vi "HFRR ADV v013 new software.vi"() -> ()   [LabVIEW 2025] (continued)
    n921 = Wait (ms)(milliseconds to wait=u32 20 ("millisecond timer value")) -> ()  [unwired: 1 out]
    n922 = local read "Quit"() -> (w1050:bool)
  }
  n923 = while {
    tunnel: w33 -> [_]
    tunnel: w17 -> [_]
    stop <- w1148 stop-if-true
    # "New Adv Logics"
    n924 = local read "Main Tab"() -> (w1128:T2)
    n925 = local read "Main Tab"() -> (w1146:T2)
    n926 = local read "Sign In"() -> (w1145:bool)
    n927 = case shown="\"Adv Scar\"" w1128 {
      frame "HOME", Default {
        n928 = local read "LIVE FEED MIN TEMP"() -> (w1281:bool)
        n929 = local write "LIVE FEED MAX TEMP"(TRUE ("LIVE FEED MAX TEMP")) -> ()
        n930 = local read "CAMERA ROI MIN TEMP"() -> (w1279:bool)
        n931 = case shown="True" w1281 {
          selector: w1281 -> [_ w1288]
          frame False {
          }
          frame True {
            n932 = Not(x=w1288) -> (.not. x?=w1287:bool)
            n933 = local write "LIVE FEED MIN TEMP"(w1287) -> ()
            n934 = call "CAMERA LIVE FEED FGV.vi"("Enum - Menu"=CAMERA_LIVE_FEED_ENUM."CAMERA MINIMIZE") -> ()  [unwired: 9 in, 2 out]
          }
        }
        n935 = case shown="True" w1279 {
          selector: w1279 -> [_ w1285]
          frame False {
          }
          frame True {
            n936 = Not(x=w1285) -> (.not. x?=w1284:bool)
            n937 = local write "CAMERA ROI MIN TEMP"(w1284) -> ()
            n938 = call "IMAGE ANALYSIS.vi"("Enum"=POST_ANALYSIS_ENUM."MINIMIZE UI") -> ()  [unwired: 9 in, 2 out]
          }
        }
        n939 = local write "CAMERA ROI MAX TEMP"(TRUE ("CAMERA ROI MAX TEMP")) -> ()
      }
      frame "Test Setup" {
        n940 = local read "LIVE FEED MIN TEMP"() -> (w1291:bool)
        n941 = local read "CAMERA ROI MIN TEMP"() -> (w1289:bool)
        n942 = local write "LIVE FEED MAX TEMP"(TRUE ("LIVE FEED MAX TEMP")) -> ()
        n943 = case shown="True" w1291 {
          selector: w1291 -> [_ w1298]
          frame False {
          }
          frame True {
            n944 = Not(x=w1298) -> (.not. x?=w1297:bool)
            n945 = local write "LIVE FEED MIN TEMP"(w1297) -> ()
            n946 = call "CAMERA LIVE FEED FGV.vi"("Enum - Menu"=CAMERA_LIVE_FEED_ENUM."CAMERA MINIMIZE") -> ()  [unwired: 9 in, 2 out]
          }
        }
        n947 = case shown="True" w1289 {
          selector: w1289 -> [_ w1295]
          frame False {
          }
          frame True {
            n948 = Not(x=w1295) -> (.not. x?=w1294:bool)
            n949 = local write "CAMERA ROI MIN TEMP"(w1294) -> ()
            n950 = call "IMAGE ANALYSIS.vi"("Enum"=POST_ANALYSIS_ENUM."MINIMIZE UI") -> ()  [unwired: 9 in, 2 out]
          }
        }
        n951 = local write "CAMERA ROI MAX TEMP"(TRUE ("CAMERA ROI MAX TEMP")) -> ()
      }
      frame "Acquire" {
        n952 = local read "LIVE FEED MIN TEMP"() -> (w1301:bool)
        n953 = local write "LIVE FEED MAX TEMP"(TRUE ("LIVE FEED MAX TEMP")) -> ()
        n954 = local read "CAMERA ROI MIN TEMP"() -> (w1299:bool)
        n955 = case shown="True" w1301 {
          selector: w1301 -> [_ w1308]
          frame False {
          }
          frame True {
            n956 = Not(x=w1308) -> (.not. x?=w1307:bool)
            n957 = local write "LIVE FEED MIN TEMP"(w1307) -> ()
            n958 = call "CAMERA LIVE FEED FGV.vi"("Enum - Menu"=CAMERA_LIVE_FEED_ENUM."CAMERA MINIMIZE") -> ()  [unwired: 9 in, 2 out]
          }
        }
        n959 = case shown="True" w1299 {
          selector: w1299 -> [_ w1305]
          frame False {
          }
          frame True {
            n960 = Not(x=w1305) -> (.not. x?=w1304:bool)
            n961 = local write "CAMERA ROI MIN TEMP"(w1304) -> ()
            n962 = call "IMAGE ANALYSIS.vi"("Enum"=POST_ANALYSIS_ENUM."MINIMIZE UI") -> ()  [unwired: 9 in, 2 out]
          }
        }
        n963 = local write "CAMERA ROI MAX TEMP"(TRUE ("CAMERA ROI MAX TEMP")) -> ()
      }
      frame "Adv Scar" {
        n964 = local read "CAMERA ROI MIN TEMP"() -> (w1309:bool)
        n965 = case shown="True" "LIVE FEED MAX TEMP" {
          selector: "LIVE FEED MAX TEMP" -> [_ w1330]
          frame False {
          }
          frame True {
            n966 = Not(x=w1330) -> (.not. x?=w1329:bool)
            n967 = local write "LIVE FEED MAX TEMP"(w1329) -> ()
            n968 = call "CAMERA LIVE FEED FGV.vi"("Enum - Menu"=CAMERA_LIVE_FEED_ENUM."CAMERA RESTORE") -> ("error out"=w1320:errorcluster)  [unwired: 9 in, 1 out]
            n969 = Type Cast(type=30, x=0) -> (*(type *) &x=w1324:i32)
            n970 = Add(x=w1324, y=48) -> (x+y=w1325:i32)
            n971 = call "CAMERA LIVE FEED FGV.vi"("Enum - Menu"=CAMERA_LIVE_FEED_ENUM."CAMERA MODE SET", "error in (no error)"=w1320, "CAMERA MODE"=w1325) -> ("error out"=w1317:errorcluster)  [unwired: 7 in, 1 out]
            n972 = call "CAMERA LIVE FEED FGV.vi"("Enum - Menu"=CAMERA_LIVE_FEED_ENUM."CAMERA GRAY", "error in (no error)"=w1317) -> ("error out"=w1316:errorcluster)  [unwired: 8 in, 1 out]
            n973 = call "LIST FILE NAMES.vi"("error in (no error)"=w1316) -> ("error out"=w1326:errorcluster, "filenames"=w1327:string[])  [unwired: 9 in]
            n974 = property on="FILE 3" class="CmbBox"(error in=w1326, "Strings[]"=w1327) -> ()  [unwired: 1 in, 2 out]
          }
        }
        n975 = case shown="True" w1309 {
          selector: w1309 -> [_ w1315]
          frame False {
          }
          frame True {
            n976 = Not(x=w1315) -> (.not. x?=w1314:bool)
            n977 = local write "CAMERA ROI MIN TEMP"(w1314) -> ()
            n978 = call "IMAGE ANALYSIS.vi"("Enum"=POST_ANALYSIS_ENUM."MINIMIZE UI") -> ()  [unwired: 9 in, 2 out]
          }
        }
        n979 = local write "CAMERA ROI MAX TEMP"(TRUE ("CAMERA ROI MAX TEMP")) -> ()
        "LIVE FEED MIN TEMP" <- TRUE ("LIVE FEED MIN TEMP")
      }
      frame "Adv Scar Report" {
        n980 = local read "CAMERA ROI MAX TEMP"() -> (w1331:bool)
        n981 = local read "LIVE FEED MIN TEMP"() -> (w1333:bool)
        n982 = local write "LIVE FEED MAX TEMP"(TRUE ("LIVE FEED MAX TEMP")) -> ()
        n983 = case shown="True" w1333 {
          selector: w1333 -> [_ w1342]
          frame False {
          }
          frame True {
            n984 = Not(x=w1342) -> (.not. x?=w1341:bool)
            n985 = local write "LIVE FEED MIN TEMP"(w1341) -> ()
            n986 = call "CAMERA LIVE FEED FGV.vi"("Enum - Menu"=CAMERA_LIVE_FEED_ENUM."CAMERA MINIMIZE") -> ()  [unwired: 9 in, 2 out]
          }
        }
        n987 = case shown="True" w1331 {
          selector: w1331 -> [_ w1339]
          frame False {
          }
          frame True {
            n988 = Not(x=w1339) -> (.not. x?=w1337:bool)
            n989 = local write "CAMERA ROI MAX TEMP"(w1337) -> ()
            n990 = call "IMAGE ANALYSIS.vi"("Enum"=POST_ANALYSIS_ENUM."SHOW UI") -> ("error out"=w1336:errorcluster)  [unwired: 9 in, 1 out]
            n991 = call "LIST FILE NAMES.vi"("error in (no error)"=w1336) -> ("filenames"=w1335:string[])  [unwired: 9 in, 1 out]
            n992 = property on="Test File List :" class="CmbBox"("Strings[]"=w1335) -> ()  [unwired: 2 in, 2 out]
          }
        }
        n993 = local write "CAMERA ROI MIN TEMP"(TRUE ("CAMERA ROI MIN TEMP")) -> ()
      }
      frame "Compare Files" {
        n994 = local read "LIVE FEED MIN TEMP"() -> (w1345:bool)
        n995 = local write "LIVE FEED MAX TEMP"(TRUE ("LIVE FEED MAX TEMP")) -> ()
        n996 = local read "CAMERA ROI MIN TEMP"() -> (w1343:bool)
        n997 = case shown="True" w1345 {
          selector: w1345 -> [_ w1352]
          frame False {
          }
          frame True {
            n998 = Not(x=w1352) -> (.not. x?=w1351:bool)
            n999 = local write "LIVE FEED MIN TEMP"(w1351) -> ()
            n1000 = call "CAMERA LIVE FEED FGV.vi"("Enum - Menu"=CAMERA_LIVE_FEED_ENUM."CAMERA MINIMIZE") -> ()  [unwired: 9 in, 2 out]
          }
        }
        n1001 = case shown="True" w1343 {
          selector: w1343 -> [_ w1349]
          frame False {
          }
          frame True {
            n1002 = Not(x=w1349) -> (.not. x?=w1348:bool)
            n1003 = local write "CAMERA ROI MIN TEMP"(w1348) -> ()
            n1004 = call "IMAGE ANALYSIS.vi"("Enum"=POST_ANALYSIS_ENUM."MINIMIZE UI") -> ()  [unwired: 9 in, 2 out]
          }
        }
        n1005 = local write "CAMERA ROI MAX TEMP"(TRUE ("CAMERA ROI MAX TEMP")) -> ()
      }
      frame "About" {
        n1006 = local read "LIVE FEED MIN TEMP"() -> (w1355:bool)
        n1007 = local write "LIVE FEED MAX TEMP"(TRUE ("LIVE FEED MAX TEMP")) -> ()
        n1008 = local read "CAMERA ROI MIN TEMP"() -> (w1354:bool)
        n1009 = case shown="True" w1355 {
          selector: w1355 -> [_ w1362]
          frame False {
          }
          frame True {
            n1010 = Not(x=w1362) -> (.not. x?=w1361:bool)
            n1011 = local write "LIVE FEED MIN TEMP"(w1361) -> ()
            n1012 = call "CAMERA LIVE FEED FGV.vi"("Enum - Menu"=CAMERA_LIVE_FEED_ENUM."CAMERA MINIMIZE") -> ()  [unwired: 9 in, 2 out]
          }
        }
        n1013 = case shown="True" w1354 {
          selector: w1354 -> [_ w1359]
          frame False {
          }
          frame True {
            n1014 = Not(x=w1359) -> (.not. x?=w1358:bool)
            n1015 = local write "CAMERA ROI MIN TEMP"(w1358) -> ()
            n1016 = call "IMAGE ANALYSIS.vi"("Enum"=POST_ANALYSIS_ENUM."MINIMIZE UI") -> ()  [unwired: 9 in, 2 out]
          }
        }
        n1017 = local write "CAMERA ROI MAX TEMP"(TRUE ("CAMERA ROI MIN TEMP")) -> ()
      }
      frame "Advance" {
        n1018 = local read "LIVE FEED MIN TEMP"() -> (w1365:bool)
        n1019 = local write "LIVE FEED MAX TEMP"(TRUE ("LIVE FEED MAX TEMP")) -> ()
        n1020 = local read "CAMERA ROI MIN TEMP"() -> (w1363:bool)
        n1021 = case shown="True" w1365 {
          selector: w1365 -> [_ w1372]
          frame False {
          }
          frame True {
            n1022 = Not(x=w1372) -> (.not. x?=w1371:bool)
            n1023 = local write "LIVE FEED MIN TEMP"(w1371) -> ()
            n1024 = call "CAMERA LIVE FEED FGV.vi"("Enum - Menu"=CAMERA_LIVE_FEED_ENUM."CAMERA MINIMIZE") -> ()  [unwired: 9 in, 2 out]
          }
        }
        n1025 = local write "CAMERA ROI MAX TEMP"(TRUE ("CAMERA ROI MAX TEMP")) -> ()
        n1026 = case shown="True" w1363 {
          selector: w1363 -> [_ w1369]
          frame False {
          }
          frame True {
            n1027 = Not(x=w1369) -> (.not. x?=w1368:bool)
            n1028 = local write "CAMERA ROI MIN TEMP"(w1368) -> ()
            n1029 = call "IMAGE ANALYSIS.vi"("Enum"=POST_ANALYSIS_ENUM."MINIMIZE UI") -> ()  [unwired: 9 in, 2 out]
          }
        }
      }
      frame "Mooha" {
        n1030 = local read "LIVE FEED MIN TEMP"() -> (w1375:bool)
        n1031 = local write "LIVE FEED MAX TEMP"(TRUE ("LIVE FEED MAX TEMP")) -> ()
        n1032 = local read "CAMERA ROI MIN TEMP"() -> (w1373:bool)
        n1033 = case shown="True" w1375 {
          selector: w1375 -> [_ w1382]
          frame False {
          }
          frame True {
            n1034 = Not(x=w1382) -> (.not. x?=w1381:bool)
            n1035 = local write "LIVE FEED MIN TEMP"(w1381) -> ()
            n1036 = call "CAMERA LIVE FEED FGV.vi"("Enum - Menu"=CAMERA_LIVE_FEED_ENUM."CAMERA MINIMIZE") -> ()  [unwired: 9 in, 2 out]
          }
        }
        n1037 = local write "CAMERA ROI MAX TEMP"(TRUE ("CAMERA ROI MAX TEMP")) -> ()
        n1038 = case shown="True" w1373 {
          selector: w1373 -> [_ w1379]
          frame False {
          }
          frame True {
            n1039 = Not(x=w1379) -> (.not. x?=w1378:bool)
            n1040 = local write "CAMERA ROI MIN TEMP"(w1378) -> ()
            n1041 = call "IMAGE ANALYSIS.vi"("Enum"=POST_ANALYSIS_ENUM."MINIMIZE UI") -> ()  [unwired: 9 in, 2 out]
          }
        }
      }
    }
    n1042 = local read "Auto Start Test"() -> (w1119:bool)
    n1043 = case shown="True" "sign in temp" {
      frame False {
      }
      frame True {
        w1155 = 1 ("y")
        n1044 = local read "USERNAME"() -> (w1161:string)
        n1045 = local read "USER ID"() -> (w1158:string)
        n1046 = call <vilib>:"Trim Whitespace.vi"("string"=w1161) -> ("trimmed string"=w1160:string)  [unwired: 1 in]
        n1047 = call <vilib>:"Trim Whitespace.vi"("string"=w1158) -> ("trimmed string"=w1159:string)  [unwired: 1 in]
        n1048 = String Length(string=w1160) -> (length=w1157:i32)
        n1049 = String Length(string=w1159) -> (length=w1156:i32)
        n1050 = Greater?(x=w1157, y=w1155) -> (0:w1154:bool)
        n1051 = Greater?(x=w1156, y=w1155) -> (0:w1153:bool)
        n1052 = And(x=w1154, y=w1153) -> (x .and. y?=w1152:bool)
        n1053 = case shown="True" w1152 {
          frame False {
            n1054 = property on="Sign In" class="Bool (strict)"("DisabledEnum"=T17."Disabled" ("Disabled")) -> ()  [unwired: 2 in, 2 out]
          }
          frame True {
            n1055 = property on="Sign In" class="Bool (strict)"("DisabledEnum"=T17."Enabled" ("Disabled")) -> ()  [unwired: 2 in, 2 out]
          }
        }
      }
    }
    n1056 = local read "Air Temperature"() -> (w1136:bool)
    n1057 = local read "Coefficient Of Friction"() -> (w1137:bool)
    n1058 = case shown="False" w1119 {
      frame False {
        n1059 = local read "Auto stop temp"() -> (w1149:bool)
        n1060 = case shown="True" w1149 {
          frame False {
          }
          frame True {
            n1061 = local write "Auto Start Temp"(FALSE ("Auto Start Temp")) -> ()
          }
        }
      }
      frame True {
        "Auto stop temp" <- TRUE ("Auto stop temp")
      }
    }
    n1062 = local read "Humidity"() -> (w1135:bool)
    n1063 = case shown="\"HOME\"" w1146 {
      frame "HOME" {
        n1064 = local write "main tab sub"(enum32{"Page 1", "Page 2"}."Page 1" ("main tab sub")) -> ()
      }
      frame Default {
        n1065 = local write "main tab sub"(enum32{"Page 1", "Page 2"}."Page 2" ("main tab sub")) -> ()
      }
    }
    n1066 = case shown="True" w1145 {
      selector: w1145 -> [_ w1496]
      frame False {
      }
      frame True {
        n1067 = Not(x=w1496) -> (.not. x?=w1495:bool)
        n1068 = local write "Sign In"(w1495) -> ()
        n1069 = local write "Main Dashboard Buttons"(T23."Test Setup" ("Main Dashboard Buttons")) -> ()
      }
    }
    n1070 = case shown="\"Numeric Display\", Default" "Num/Graph" {
      frame "Numeric Display", Default {
        n1071 = property on="Single/Multiple" class="RadioBtnsControl (strict)"("Visible"=FALSE) -> ()  [unwired: 2 in, 2 out]
        n1072 = property on="Single - Graph" class="Ring (strict)"("Visible"=FALSE) -> ()  [unwired: 2 in, 2 out]
        n1073 = local write "Main Tab Display"(T4."Dashboard 1" ("Main Tab Display")) -> ()
      }
      frame "Graph Display" {
        n1074 = property on="Single/Multiple" class="RadioBtnsControl (strict)"("Visible"=TRUE) -> ()  [unwired: 2 in, 2 out]
        n1075 = case shown="\"Multiple\"" "Single/Multiple" {
          frame "Single ", Default {
            n1076 = property on="Single - Graph" class="Ring (strict)"("Visible"=TRUE) -> ()  [unwired: 2 in, 2 out]
            n1077 = local write "Main Tab Display"(T4."Dashboard 3" ("Main Tab Display")) -> ()
          }
          frame "Multiple" {
            n1078 = property on="Single - Graph" class="Ring (strict)"("Visible"=FALSE) -> ()  [unwired: 2 in, 2 out]
            n1079 = local write "Main Tab Display"(T4."Dashboard 2" ("Main Tab Display")) -> ()
          }
        }
      }
    }
    n1080 = local read "Stroke"() -> (w1134:bool)
    n1081 = local read "USERNAME"() -> (w1140:string)
    n1082 = local read "USER ID"() -> (w1139:string)
    n1083 = case shown="True" w1137 {
      selector: w1137 -> [_ w1422]
      frame False {
      }
      frame True {
        n1084 = Not(x=w1422) -> (.not. x?=w1421:bool)
        n1085 = local write "Coefficient Of Friction"(w1421) -> ()
        n1086 = local write "Tab Control 2"(T6."Coefficient Of Friction" ("Tab Control 2")) -> ()
      }
    }
    n1087 = case shown="True" w1136 {
      selector: w1136 -> [_ w1419]
      frame False {
      }
      frame True {
        n1088 = Not(x=w1419) -> (.not. x?=w1417:bool)
        n1089 = local write "Air Temperature"(w1417) -> ()
        n1090 = local write "Tab Control 2"(T6."Air Temperature" ("Tab Control 2")) -> ()
      }
    }
    n1091 = local write "Operator ID"(w1139) -> ()
    n1092 = case shown="True" w1134 {
      selector: w1134 -> [_ w1413]
      frame False {
      }
      frame True {
        n1093 = Not(x=w1413) -> (.not. x?=w1411:bool)
        n1094 = local write "Stroke"(w1411) -> ()
        n1095 = local write "Tab Control 2"(T6."Stroke" ("Tab Control 2")) -> ()
      }
    }
    n1096 = local write "tested by"(w1140) -> ()
    n1097 = case shown="True" w1135 {
      selector: w1135 -> [_ w1416]
      frame False {
      }
      frame True {
        n1098 = Not(x=w1416) -> (.not. x?=w1414:bool)
        n1099 = local write "Humidity"(w1414) -> ()
        n1100 = local write "Tab Control 2"(T6."Humidity" ("Tab Control 2")) -> ()
      }
    }
    n1101 = case shown="\"Calibration\"" "Main Dashboard Buttons" {
      tunnel: [T2."HOME" ("Main Tab") T2."Test Setup" ("Main Tab") T2."Acquire" ("Main Tab") T2."Adv Scar" ("Main Tab") T2."Adv Scar Report" ("Main Tab") T2."Compare Files" ("Main Tab") T2."Calibration" ("Main Tab") T2."About" ("Main Tab") T2."Advance" ("Main Tab")] -> w1118
      frame "Home", Default {
      }
      frame "Test Setup" {
      }
      frame "Dashboard" {
      }
      frame "Imaging" {
      }
      frame "Report" {
      }
      frame "Analysis" {
      }
      frame "Calibration" {
      }
      frame "About" {
      }
      frame "Advance" {
      }
    }
    n1102 = Wait (ms)(milliseconds to wait=u32 100) -> ()  [unwired: 1 out]
    n1103 = local read "Main Tab Display"() -> (w1138:T4)
    n1104 = local write "Main Tab"(w1118) -> ()
    n1105 = case shown="\"Dashboard 3\"" w1138 {
      frame "Dashboard 1", Default {
        n1106 = property on="Reset Graph" class="Bool (strict)"("Visible"=FALSE) -> ()  [unwired: 2 in, 2 out]
      }
      frame "Dashboard 2" {
        n1107 = property on="Reset Graph" class="Bool (strict)"("Visible"=TRUE) -> ()  [unwired: 2 in, 2 out]
      }
      frame "Dashboard 3" {
        n1108 = property on="Reset Graph" class="Bool (strict)"("Visible"=TRUE) -> ()  [unwired: 2 in, 2 out]
      }
    }
    n1109 = local read "SCAR MEASURMENT"() -> (w1126:enum32{"Auto Scar", "Manual Scar"})
    n1110 = local read "Humidity"() -> (w1141:bool)
    n1111 = local read "Cap Live Image"() -> (w1123:bool)
    n1112 = local read "Sample Temperature"() -> (w1133:bool)
    n1113 = local read "Air Temp vs Humidity"() -> (w1131:bool)
    n1114 = local read "Frequency"() -> (w1132:bool)
    n1115 = case shown="True" w1141 {
      frame False {
        n1116 = local write "Humidity On Command"(TRUE ("Humidity On Command")) -> ()
        n1117 = case shown="True" "Humidity Off Command" {
          selector: "Humidity Off Command" -> [_ w1429]
          frame False {
          }
          frame True {
            n1118 = stacked-sequence {
              frame #0 {
                n1119 = local read "WriteHumidity"() -> (w1431:string[])
                n1120 = Insert Into Array(array=w1431, new element="R;1" ("new element/subarray")) -> (w1432:string[])  [unwired: 1 in]
                n1121 = local write "WriteHumidity"(w1432) -> ()
              }
              frame #1 {
                n1122 = Wait (ms)(milliseconds to wait=u32 2000) -> ()  [unwired: 1 out]
              }
              frame #2 {
                n1123 = local read "EVENT LOG"() -> (w1438:string)
                n1124 = local read "WriteHumidity"() -> (w1435:string[])
                n1125 = call "Event Log.vi"("Content"="Humidity Control Off" ("string"), "EVENT LOG"=w1438) -> ("EVENT LOG"=w1439:string)  [unwired: 8 in, 1 out]
                n1126 = local write "EVENT LOG"(w1439) -> ()
                n1127 = Insert Into Array(array=w1435, new element="R;1" ("new element/subarray")) -> (w1436:string[])  [unwired: 1 in]
                n1128 = local write "WriteHumidity"(w1436) -> ()
              }
            }
            n1129 = Not(x=w1429) -> (.not. x?=w1428:bool)
            n1130 = local write "Humidity Off Command"(w1428) -> ()
          }
        }
      }
      frame True {
        n1131 = local write "Humidity Off Command"(TRUE ("Humidity Off Command")) -> ()
        n1132 = case shown="True" "Humidity On Command" {
          selector: "Humidity On Command" -> [_ w1443]
          frame False {
          }
          frame True {
            n1133 = stacked-sequence {
              frame #0 {
                n1134 = local read "Set Rh"() -> (w1449:dbl)
                n1135 = Number To Fractional String(number=w1449, precision (6)=i16 2) -> (F-format string=w1450:string)  [unwired: 2 in]
                n1136 = local read "WriteHumidity"() -> (w1447:string[])
                n1137 = Concatenate Strings("M;" ("new element/subarray"), w1450) -> (w1448:string)
                n1138 = Insert Into Array(array=w1447, new element=w1448) -> (w1446:string[])  [unwired: 1 in]
                n1139 = local write "WriteHumidity"(w1446) -> ()
              }
              frame #1 {
                n1140 = Wait (ms)(milliseconds to wait=u32 2000) -> ()  [unwired: 1 out]
              }
              frame #2 {
                n1141 = local read "Set Rh"() -> (w1457:dbl)
                n1142 = Number To Fractional String(number=w1457, precision (6)=i16 2) -> (F-format string=w1458:string)  [unwired: 2 in]
                n1143 = local read "WriteHumidity"() -> (w1455:string[])
                n1144 = Concatenate Strings("M;" ("new element/subarray"), w1458) -> (w1456:string)
                n1145 = Insert Into Array(array=w1455, new element=w1456) -> (w1454:string[])  [unwired: 1 in]
                n1146 = local write "WriteHumidity"(w1454) -> ()
              }
              frame #3 {
                n1147 = Wait (ms)(milliseconds to wait=u32 1500) -> ()  [unwired: 1 out]
              }
              frame #4 {
                (unwired) "% RH" ("string")
                (unwired) i16 2 ("precision (6)")
                (unwired) "M;" ("new element/subarray")
                n1148 = local read "Set Rh"() -> (w1465:dbl)
                n1149 = Number To Fractional String(number=w1465, precision (6)=i16 2) -> (F-format string=w1462:string)  [unwired: 2 in]
                n1150 = local read "WriteHumidity"() -> (w1467:string[])
                n1151 = Concatenate Strings("M;" ("new element/subarray"), w1462) -> (w1466:string)
                n1152 = Concatenate Strings("Humidity Set to : " ("string"), w1462, "% RH" ("string")) -> (w1460:string)
                n1153 = Insert Into Array(array=w1467, new element=w1466) -> (w1468:string[])  [unwired: 1 in]
                n1154 = disable-structure shown="Enabled" {
                  frame Enabled {
                    n1155 = local read "EVENT LOG"() -> (w1471:string)
                    n1156 = call "Event Log.vi"("Content"="Humidity Control On", "EVENT LOG"=w1471) -> ("EVENT LOG"=w1472:string)  [unwired: 8 in, 1 out]
                    n1157 = local write "EVENT LOG"(w1472) -> ()
                  }
                  frame Disabled {
                  }
                }
                n1158 = disable-structure shown="Enabled" {
                  disable-tunnel: w1460 -> [_ _]
                  frame Enabled {
                    n1159 = local read "EVENT LOG"() -> (w1474:string)
                    n1160 = call "Event Log.vi"("Content"="Humidity Control On", "EVENT LOG"=w1474) -> ("EVENT LOG"=w1475:string)  [unwired: 8 in, 1 out]
                    n1161 = local write "EVENT LOG"(w1475) -> ()
                  }
                  frame Disabled {
                  }
                }
                n1162 = local write "WriteHumidity"(w1468) -> ()
              }
            }
            n1163 = Not(x=w1443) -> (.not. x?=w1442:bool)
            n1164 = local write "Humidity On Command"(w1442) -> ()
          }
        }
      }
    }
    n1165 = Equal?(x=w1126, y=enum32{"Auto Scar", "Manual Scar"}."Auto Scar" ("SCAR MEASURMENT")) -> (x = y?=w1122:bool)
    n1166 = local read "TEST STANDARD"() -> (w1129:T3)
    n1167 = And(x=w1123, y=w1122) -> (x .and. y?=w1124:bool)
    n1168 = case shown="True" w1124 {
      selector: w1124 -> [_ w1228]
      tunnel: errorcluster {"status"=FALSE, "code"=0, "source"=""} ("error in (no error) 3") -> [_ w1229]
      frame False {
      }
      frame True {
        n1169 = stacked-sequence {
          tunnel: w1229 -> [_ _ _ _ _ _ _ w1277]
          tunnel: w1228 -> [_ _ _ _ _ w1258 _ _]
          frame #0 {
            n1170 = call "CAMERA LIVE FEED FGV.vi"("Enum - Menu"=CAMERA_LIVE_FEED_ENUM."CAMERA MINIMIZE") -> ()  [unwired: 9 in, 2 out]
          }
          frame #1 {
            n1171 = property on="Auto Scar Check  2" class="Clust (strict)"("Visible"=TRUE) -> ()  [unwired: 2 in, 2 out]
          }
          frame #2 {
            n1172 = String To Path(string="C:\\LAB-IQ\\Image Calibrate v01.dcf") -> (path=w1234:path)
            n1173 = Open/Create/Replace File ("Open File")(file path (use dialog)=w1234) -> (refnum out=w1235:refnum<file>)  [unwired: 5 in, 2 out]
            n1174 = for {
              N: 4 -> [_]
              tunnel: w1235 -> [w1241]
              i -> [w1237]
              n1175 = Read from Text File ("Read File")(file (use dialog)=w1241) -> (text=w1242:string)  [unwired: 3 in, 3 out]
              n1176 = String Subset(string=w1242, offset (0)=6, length (rest)=10 ("length (rest)")) -> (substring=w1238:string)
              n1177 = Fract/Exp String To Number(string=w1238) -> (number=w1236:dbl)  [unwired: 3 in, 1 out]
              n1178 = case shown="0" w1237 {
                tunnel: w1236 -> [w1243 w1244 _ w1245 _]
                frame 0 {
                  "5x Gain" <- w1243
                }
                frame 1 {
                  "10x Gain" <- w1244
                }
                frame 2 {
                }
                frame 3 {
                  "100x gain" <- w1245
                }
                frame 4, Default {
                }
              }
            }
          }
          frame #3 {
            n1179 = local read "FILE 3"() -> (w1251:string)
            n1180 = call <vilib>:"Trim Whitespace.vi"("string"="C:\\LAB-IQ\\images\\") -> ("trimmed string"=w1253:string)  [unwired: 1 in]
            n1181 = String To Path(string=w1253) -> (path=w1252:path)
            n1182 = Concatenate Strings(w1251, ".png" ("string")) -> (w1250:string)
            n1183 = Build Path(base path=w1252, name or relative path=w1250) -> (appended path=w1248:path)
            "Image path" <- w1248
            n1184 = Path To String(path=w1248) -> (string=w1247:string)
            n1185 = call "CAMERA LIVE FEED FGV.vi"("Enum - Menu"=CAMERA_LIVE_FEED_ENUM."CAMERA SAVE", "Image Path"=w1247) -> ()  [unwired: 8 in, 2 out]
          }
          frame #4 {
            n1186 = One Button Dialog(message="Image saved successfully") -> ()  [unwired: 1 in, 1 out]
          }
          frame #5 {
            n1187 = local read "TEST STANDARD"() -> (w1257:T3)
            n1188 = local read "Magnification len live scar"() -> (w1269:string)
            n1189 = Not(x=w1258) -> (.not. x?=w1259:bool)
            n1190 = local write "Cap Live Image"(w1259) -> ()
            n1191 = case shown="\"ISO 12156\"" w1257 {
              tunnel: ["ASTM D6079" "ISO 12156"] -> w1256
              frame "ASTM D6079", Default {
              }
              frame "ISO 12156" {
              }
            }
            n1192 = case shown="\"5x\", Default" w1269 {
              tunnel: [w1272 w1273] -> w1268
              frame "5x", Default {
                n1193 = local read "5x Gain"() -> (w1272:dbl)
              }
              frame "10x" {
                # "5x"
                n1194 = local read "10x Gain"() -> (w1273:dbl)
              }
            }
            n1195 = local read "Image path"() -> (w1267:path)
            n1196 = local read "FILE 3"() -> (w1260:string)
            n1197 = call "EDGE DETCTION.vi"("GAIN VALUE"=w1268, "Image Path"=w1267) -> ("error out"=w1266:errorcluster, "return value"=w1265:cluster{string, string, dbl, dbl, dbl})  [unwired: 8 in]
            n1198 = Bundle By Name(cluster=T24 {"File Name"="", "Test Method"="", "Operator"="", "Fuel Description"="", "Date and time"=""} ("Main Ref"), "File Name"=w1260, "Test Method"=w1256) -> (w1261:T24)
            n1199 = call "duf file read.vi"("error in (no error)"=w1266, "Main Ref"=w1261) -> ("error out"=w1264:errorcluster, "Main Ref 2"=w1262:T24)  [unwired: 8 in]
            n1200 = call "EDGE DETECTION REPORT.vi"("error in (no error)"=w1264, "return value 2"=w1265, "Main Ref"=w1262) -> ()  [unwired: 8 in, 1 out]
          }
          frame #6 {
            n1201 = property on="Auto Scar Check  2" class="Clust (strict)"("Visible"=FALSE) -> ()  [unwired: 2 in, 2 out]
          }
          frame #7 {
            n1202 = call "CAMERA LIVE FEED FGV.vi"("Enum - Menu"=CAMERA_LIVE_FEED_ENUM."CAMERA MINIMIZE", "error in (no error)"=w1277) -> ()  [unwired: 8 in, 2 out]
            n1203 = local write "Main Dashboard Buttons"(T1."Home" ("Main Dashboard Buttons")) -> ()
            n1204 = local write "Main Tab"(T2."HOME" ("Main Tab")) -> ()
          }
        }
      }
    }
    n1205 = local read "Heater Button"() -> (w1130:bool)
    n1206 = case shown="True" w1132 {
      selector: w1132 -> [_ w1407]
      frame False {
      }
      frame True {
        n1207 = Not(x=w1407) -> (.not. x?=w1405:bool)
        n1208 = local write "Frequency"(w1405) -> ()
        n1209 = local write "Tab Control 2"(T6."Frequency" ("Tab Control 2")) -> ()
      }
    }
    n1210 = case shown="True" w1131 {
      selector: w1131 -> [_ w1404]
      frame False {
      }
      frame True {
        n1211 = Not(x=w1404) -> (.not. x?=w1402:bool)
        n1212 = local write "Air Temp vs Humidity"(w1402) -> ()
        n1213 = local write "Tab Control 2"(T6."Air Temp vs Rh" ("Tab Control 2")) -> ()
      }
    }
    n1214 = case shown="True" w1133 {
      selector: w1133 -> [_ w1410]
      frame False {
      }
      frame True {
        n1215 = Not(x=w1410) -> (.not. x?=w1408:bool)
        n1216 = local write "Sample Temperature"(w1408) -> ()
        n1217 = local write "Tab Control 2"(T6."Sample Temperature" ("Tab Control 2")) -> ()
      }
    }
    n1218 = case shown="\"Custom\"" w1129 {
      frame "ASTM D6079", Default {
        w1383 = "ASTM D6079 TEST CONDITIONS" ("Standard 2")
        n1219 = local write "Standard 2"(w1383) -> ()
        n1220 = local write "Standard"(w1383) -> ()
      }
      frame "ISO 12156" {
        w1384 = "ISO 12156 TEST CONDITIONS" ("Standard 2")
        n1221 = local write "Standard 2"(w1384) -> ()
        n1222 = local write "Standard"(w1384) -> ()
      }
      frame "CEC F-096-A-06" {
        w1385 = "CEC F-096-A-06 TEST CONDITIONS" ("Standard 2")
        n1223 = local write "Standard 2"(w1385) -> ()
        n1224 = local write "Standard"(w1385) -> ()
      }
      frame "Custom" {
        w1386 = "CUSTOM TEST CONDITIONS" ("Standard 2")
        n1225 = local write "Standard 2"(w1386) -> ()
        n1226 = local write "Standard"(w1386) -> ()
      }
    }
    n1227 = case shown="True" w1130 {
      frame False {
        n1228 = local write "Temperature On Command"(TRUE ("Temperature On Command")) -> ()
        n1229 = case shown="True" "Temperature Off Command" {
          selector: "Temperature Off Command" -> [_ w1390]
          frame False {
          }
          frame True {
            n1230 = Not(x=w1390) -> (.not. x?=w1389:bool)
            n1231 = local read "EVENT LOG"() -> (w1393:string)
            n1232 = local write "Temperature Off Command"(w1389) -> ()
            n1233 = call "Event Log.vi"("Content"="Heater Off", "EVENT LOG"=w1393) -> ("EVENT LOG"=w1392:string)  [unwired: 8 in, 1 out]
            n1234 = local write "EVENT LOG"(w1392) -> ()
          }
        }
      }
      frame True {
        n1235 = local write "Temperature Off Command"(TRUE ("Temperature Off Command")) -> ()
        n1236 = case shown="True" "Temperature On Command" {
          selector: "Temperature On Command" -> [_ w1397]
          frame False {
          }
          frame True {
            n1237 = Not(x=w1397) -> (.not. x?=w1396:bool)
            n1238 = local write "Temperature On Command"(w1396) -> ()
            n1239 = disable-structure shown="Enabled" {
              disable-tunnel: "Heater On" -> [w1399 _]
              frame Enabled {
                n1240 = local read "EVENT LOG"() -> (w1400:string)
                n1241 = call "Event Log.vi"("Content"=w1399, "EVENT LOG"=w1400) -> ("EVENT LOG"=w1401:string)  [unwired: 8 in, 1 out]
                n1242 = local write "EVENT LOG"(w1401) -> ()
              }
              frame Disabled {
              }
            }
          }
        }
      }
    }
    n1243 = local read "Main Tab"() -> (w1121:T2)
    n1244 = case shown="\"About\"" w1121 {
      frame "HOME", Default {
        w1164 = T17."Enabled" ("Disabled")
        n1245 = local read "Service Password enable"() -> (w1166:bool)
        n1246 = property on="Imaging" class="Bool (strict)"("DisabledEnum"=w1164) -> ()  [unwired: 2 in, 2 out]
        n1247 = property on="Dashboard" class="Bool (strict)"("DisabledEnum"=w1164) -> ()  [unwired: 2 in, 2 out]
        n1248 = property on="Test Setup" class="Bool (strict)"("DisabledEnum"=w1164) -> ()  [unwired: 2 in, 2 out]
        n1249 = property on="Analysis" class="Bool (strict)"("DisabledEnum"=w1164) -> ()  [unwired: 2 in, 2 out]
        n1250 = property on="Home" class="Bool (strict)"("DisabledEnum"=w1164) -> ()  [unwired: 2 in, 2 out]
        n1251 = property on="Report" class="Bool (strict)"("DisabledEnum"=w1164) -> ()  [unwired: 2 in, 2 out]
        n1252 = property on="Main Dashboard Buttons" class="RadioBtnsControl (strict)"("DisabledEnum"=w1164) -> ()  [unwired: 2 in, 2 out]
        n1253 = property on="Calibration" class="Bool (strict)"("DisabledEnum"=w1164) -> ()  [unwired: 2 in, 2 out]
        n1254 = case shown="True" w1166 {
          tunnel: [T17."Disabled" ("Disabled") T17."Enabled" ("Disabled")] -> w1165
          frame False {
          }
          frame True {
          }
        }
        n1255 = property on="About" class="Bool (strict)"("DisabledEnum"=w1165) -> ()  [unwired: 2 in, 2 out]
      }
      frame "Test Setup" {
        w1171 = T17."Enabled" ("Disabled")
        n1256 = local read "Service Password enable"() -> (w1170:bool)
        n1257 = property on="Dashboard" class="Bool (strict)"("DisabledEnum"=T17."Disabled" ("Disabled")) -> ()  [unwired: 2 in, 2 out]
        n1258 = property on="Imaging" class="Bool (strict)"("DisabledEnum"=w1171) -> ()  [unwired: 2 in, 2 out]
        n1259 = property on="Analysis" class="Bool (strict)"("DisabledEnum"=w1171) -> ()  [unwired: 2 in, 2 out]
        n1260 = property on="Home" class="Bool (strict)"("DisabledEnum"=w1171) -> ()  [unwired: 2 in, 2 out]
        n1261 = property on="Report" class="Bool (strict)"("DisabledEnum"=w1171) -> ()  [unwired: 2 in, 2 out]
        n1262 = property on="Test Setup" class="Bool (strict)"("DisabledEnum"=w1171) -> ()  [unwired: 2 in, 2 out]
        n1263 = case shown="True" w1170 {
          tunnel: [T17."Disabled" ("Disabled") T17."Enabled" ("Disabled")] -> w1169
          frame False {
          }
          frame True {
          }
        }
        n1264 = property on="About" class="Bool (strict)"("DisabledEnum"=w1169) -> ()  [unwired: 2 in, 2 out]
      }
      frame "Adv Scar" {
        w1178 = T17."Enabled" ("Disabled")
        n1265 = property on="Dashboard" class="Bool (strict)"("DisabledEnum"=T17."Disabled" ("Disabled")) -> ()  [unwired: 2 in, 2 out]
        n1266 = property on="Imaging" class="Bool (strict)"("DisabledEnum"=w1178) -> ()  [unwired: 2 in, 2 out]
        n1267 = property on="Analysis" class="Bool (strict)"("DisabledEnum"=w1178) -> ()  [unwired: 2 in, 2 out]
        n1268 = property on="Home" class="Bool (strict)"("DisabledEnum"=w1178) -> ()  [unwired: 2 in, 2 out]
        n1269 = property on="Report" class="Bool (strict)"("DisabledEnum"=w1178) -> ()  [unwired: 2 in, 2 out]
        n1270 = property on="Test Setup" class="Bool (strict)"("DisabledEnum"=w1178) -> ()  [unwired: 2 in, 2 out]
        n1271 = local read "Service Password enable"() -> (w1176:bool)
        n1272 = case shown="True" w1176 {
          tunnel: [T17."Disabled" ("Disabled") T17."Enabled" ("Disabled")] -> w1175
          frame False {
          }
          frame True {
          }
        }
        n1273 = property on="About" class="Bool (strict)"("DisabledEnum"=w1175) -> ()  [unwired: 2 in, 2 out]
      }
      frame "Calibration" {
        w1181 = T17."Enabled" ("Disabled")
        n1274 = property on="Dashboard" class="Bool (strict)"("DisabledEnum"=T17."Disabled" ("Disabled")) -> ()  [unwired: 2 in, 2 out]
        n1275 = property on="Imaging" class="Bool (strict)"("DisabledEnum"=w1181) -> ()  [unwired: 2 in, 2 out]
        n1276 = property on="Analysis" class="Bool (strict)"("DisabledEnum"=w1181) -> ()  [unwired: 2 in, 2 out]
        n1277 = property on="Home" class="Bool (strict)"("DisabledEnum"=w1181) -> ()  [unwired: 2 in, 2 out]
        n1278 = property on="Report" class="Bool (strict)"("DisabledEnum"=w1181) -> ()  [unwired: 2 in, 2 out]
        n1279 = property on="Test Setup" class="Bool (strict)"("DisabledEnum"=w1181) -> ()  [unwired: 2 in, 2 out]
        n1280 = local read "Service Password enable"() -> (w1183:bool)
        n1281 = property on="Calibration" class="Bool (strict)"("DisabledEnum"=w1181) -> ()  [unwired: 2 in, 2 out]
        n1282 = case shown="True" w1183 {
          tunnel: [T17."Disabled" ("Disabled") T17."Enabled" ("Disabled")] -> w1182
          frame False {
          }
          frame True {
          }
        }
        n1283 = property on="About" class="Bool (strict)"("DisabledEnum"=w1182) -> ()  [unwired: 2 in, 2 out]
      }
      frame "Adv Scar Report" {
        w1189 = T17."Enabled" ("Disabled")
        n1284 = property on="Dashboard" class="Bool (strict)"("DisabledEnum"=T17."Disabled" ("Disabled")) -> ()  [unwired: 2 in, 2 out]
        n1285 = property on="Imaging" class="Bool (strict)"("DisabledEnum"=w1189) -> ()  [unwired: 2 in, 2 out]
        n1286 = property on="Analysis" class="Bool (strict)"("DisabledEnum"=w1189) -> ()  [unwired: 2 in, 2 out]
        n1287 = property on="Home" class="Bool (strict)"("DisabledEnum"=w1189) -> ()  [unwired: 2 in, 2 out]
        n1288 = property on="Report" class="Bool (strict)"("DisabledEnum"=w1189) -> ()  [unwired: 2 in, 2 out]
        n1289 = property on="Test Setup" class="Bool (strict)"("DisabledEnum"=w1189) -> ()  [unwired: 2 in, 2 out]
        n1290 = local read "Service Password enable"() -> (w1188:bool)
        n1291 = case shown="True" w1188 {
          tunnel: [T17."Disabled" ("Disabled") T17."Enabled" ("Disabled")] -> w1187
          frame False {
          }
          frame True {
          }
        }
        n1292 = property on="About" class="Bool (strict)"("DisabledEnum"=w1187) -> ()  [unwired: 2 in, 2 out]
      }
      frame "Compare Files" {
        w1195 = T17."Enabled" ("Disabled")
        n1293 = local read "Service Password enable"() -> (w1194:bool)
        n1294 = property on="Dashboard" class="Bool (strict)"("DisabledEnum"=T17."Disabled" ("Disabled")) -> ()  [unwired: 2 in, 2 out]
        n1295 = property on="Imaging" class="Bool (strict)"("DisabledEnum"=w1195) -> ()  [unwired: 2 in, 2 out]
        n1296 = property on="Analysis" class="Bool (strict)"("DisabledEnum"=w1195) -> ()  [unwired: 2 in, 2 out]
        n1297 = property on="Home" class="Bool (strict)"("DisabledEnum"=w1195) -> ()  [unwired: 2 in, 2 out]
        n1298 = property on="Report" class="Bool (strict)"("DisabledEnum"=w1195) -> ()  [unwired: 2 in, 2 out]
        n1299 = property on="Test Setup" class="Bool (strict)"("DisabledEnum"=w1195) -> ()  [unwired: 2 in, 2 out]
        n1300 = case shown="True" w1194 {
          tunnel: [T17."Disabled" ("Disabled") T17."Enabled" ("Disabled")] -> w1193
          frame False {
          }
          frame True {
          }
        }
        n1301 = property on="About" class="Bool (strict)"("DisabledEnum"=w1193) -> ()  [unwired: 2 in, 2 out]
      }
      frame "Acquire" {
        n1302 = local read "Service Password enable"() -> (w1200:bool)
        n1303 = property on="Test Setup" class="Bool (strict)"("DisabledEnum"=T17."Disabled" ("Disabled")) -> ()  [unwired: 2 in, 2 out]
        n1304 = local read "Auto Start Test"() -> (w1202:bool)
        n1305 = local read "RUN"() -> (w1204:bool)
        n1306 = case shown="True" w1200 {
          tunnel: [T17."Disabled" ("Disabled") T17."Enabled" ("Disabled")] -> w1201
          frame False {
          }
          frame True {
          }
        }
        n1307 = Or(x=w1204, y=w1202) -> (x .or. y?=w1203:bool)
        n1308 = case shown="True" w1203 {
          tunnel: [T17."Enabled" ("Disabled") T17."Disabled" ("Disabled")] -> w1199
          frame False {
          }
          frame True {
          }
        }
        n1309 = property on="About" class="Bool (strict)"("DisabledEnum"=w1201) -> ()  [unwired: 2 in, 2 out]
        n1310 = property on="Imaging" class="Bool (strict)"("DisabledEnum"=w1199) -> ()  [unwired: 2 in, 2 out]
        n1311 = property on="Dashboard" class="Bool (strict)"("DisabledEnum"=w1199) -> ()  [unwired: 2 in, 2 out]
        n1312 = property on="Analysis" class="Bool (strict)"("DisabledEnum"=w1199) -> ()  [unwired: 2 in, 2 out]
        n1313 = property on="Home" class="Bool (strict)"("DisabledEnum"=w1199) -> ()  [unwired: 2 in, 2 out]
        n1314 = property on="Report" class="Bool (strict)"("DisabledEnum"=w1199) -> ()  [unwired: 2 in, 2 out]
        n1315 = property on="Calibration" class="Bool (strict)"("DisabledEnum"=w1199) -> ()  [unwired: 2 in, 2 out]
      }
      frame "About" {
        n1316 = local read "FILE"() -> (w1218:string)
        n1317 = local read "TEST FILE NAM,E SAVED"() -> (w1211:bool)
        n1318 = call <vilib>:"Trim Whitespace.vi"("string"=w1218) -> ("trimmed string"=w1217:string)  [unwired: 1 in]
        n1319 = local read "Auto Start Test"() -> (w1221:bool)
        n1320 = String Length(string=w1217) -> (length=w1216:i32)
        n1321 = Greater?(x=w1216, y=1) -> (0:w1213:bool)
        n1322 = And(x=w1213, y=w1211) -> (x .and. y?=w1212:bool)
        n1323 = local read "RUN"() -> (w1223:bool)
        n1324 = case shown="True" w1212 {
          tunnel: [T17."Disabled" ("Disabled") T17."Enabled" ("Disabled")] -> w1214
          frame False {
          }
          frame True {
          }
        }
        n1325 = Or(x=w1223, y=w1221) -> (x .or. y?=w1222:bool)
        n1326 = property on="About" class="Bool (strict)"("DisabledEnum"=T17."Enabled" ("Disabled")) -> ()  [unwired: 2 in, 2 out]
        n1327 = case shown="False" w1222 {
          tunnel: [T17."Enabled" ("Disabled") T17."Disabled" ("Disabled")] -> w1220
          frame False {
          }
          frame True {
          }
        }
        n1328 = property on="Dashboard" class="Bool (strict)"("DisabledEnum"=w1214) -> ()  [unwired: 2 in, 2 out]
        n1329 = property on="Test Setup" class="Bool (strict)"("DisabledEnum"=T17."Disabled" ("Disabled")) -> ()  [unwired: 2 in, 2 out]
        n1330 = property on="Imaging" class="Bool (strict)"("DisabledEnum"=w1220) -> ()  [unwired: 2 in, 2 out]
        n1331 = property on="Analysis" class="Bool (strict)"("DisabledEnum"=w1220) -> ()  [unwired: 2 in, 2 out]
        n1332 = property on="Home" class="Bool (strict)"("DisabledEnum"=w1220) -> ()  [unwired: 2 in, 2 out]
        n1333 = property on="Report" class="Bool (strict)"("DisabledEnum"=w1220) -> ()  [unwired: 2 in, 2 out]
      }
    }
    n1334 = local read "Quit"() -> (w1148:bool)
    "Single" <- "Single - Graph"
  }
  n1335 = disable-structure shown="Disabled" {
    disable-tunnel: [w1500 _] -> w39
    disable-tunnel: _ -> [w1499 _]
    frame Disabled {
      n1336 = while {
        tunnel: w1499 -> [_]
        tunnel: [w1501] -> w1500
        tunnel: [w1502] -> _
        i -> [w1502]
        stop <- w1501 stop-if-true
        w1518 = u16 10 items=["1.0"=10, "1.5"=15, "2.0"=20] ("stop bits (10: 1 bit)")
        n1337 = Wait (ms)(milliseconds to wait=u32 10) -> ()  [unwired: 1 out]
        n1338 = call-poly "VISA Configure Serial Port"("VISA resource name"=refnum<visa-resource-name> "ASRL1::INSTR" ("COM PORT"), "timeout (10sec)"=u32 10, "baud rate (9600)"=u32 57600, "data bits (8)"=u16 8, "stop bits (10: 1 bit)"=w1518) -> ("VISA resource name out"=w1504:refnum<visa-resource-name>, "error out"=w1513:errorcluster)  [unwired: 9 in]
        n1339 = VISA Read(VISA resource name=w1504, byte count=u32 2 ("byte count (0)")) -> (read buffer=w1512:string)  [unwired: 1 in, 3 out]
        n1340 = String Subset(string=w1512, offset (0)=0, length (rest)=2 ("length (rest)")) -> (substring=w1511:string)
        n1341 = Match Pattern(string=w1511, regular expression="<>") -> (offset past match=w1508:i32)  [unwired: 1 in, 3 out]
        n1342 = Greater Or Equal?(x=w1508, y=0) -> (x >= y?=w1503:bool)
        n1343 = case shown="True" w1503 {
          tunnel: w1504 -> [_ w1522]
          tunnel: w1513 -> [_ w1521]
          frame False {
          }
          frame True {
            n1344 = VISA Read(VISA resource name=w1522, byte count=u32 32 ("byte count (0)"), error in (no error)=w1521) -> (read buffer=w1520:string)  [unwired: 3 out]
            n1345 = String Subset(string=w1520, offset (0)=0, length (rest)=8 ("length (rest)")) -> (substring=w1524:string)
            n1346 = String Subset(string=w1520, offset (0)=8, length (rest)=8 ("length (rest)")) -> (substring=w1525:string)
            n1347 = Decimal String To Number(string=w1525) -> (number=w1532:i32)  [unwired: 2 in, 1 out]
            n1348 = Decimal String To Number(string=w1524) -> (number=w1528:i32)  [unwired: 2 in, 1 out]
            n1349 = Divide(x=w1532, y=10000) -> ()  [unwired: 1 out]
            n1350 = Divide(x=w1528, y=1000000) -> ()  [unwired: 1 out]
          }
        }
        n1351 = local read "Quit"() -> (w1501:bool)
      }
    }
    frame Enabled {
    }
  }
  n1352 = while {
    shift-right: [w1547] -> w52
    shift-left: _ -> [w1538]
    shift-right: [w1546] -> w51
    shift-left: errorcluster {"status"=TRUE, "code"=0, "source"="Init"} ("error IO") -> [w1540]
    tunnel: [w1535] -> w42
    tunnel: [w1545] -> _
    i -> [w1545]
    stop <- w1535 stop-if-true
    n1353 = local read "Port 1a"() -> (w1541:bool)
    n1354 = local read "Port 3"() -> (w1542:bool)
    n1355 = local read "Com Port 1"() -> (w1539:refnum<visa-resource-name>)
    n1356 = Or(x=w1542, y=w1541) -> (x .or. y?=w1544:bool)
    n1357 = Unbundle(w1540) -> ("status"=→"Port 3":bool)  [unwired: 2 out]
    n1358 = Not Equal?(x=w1539, y=w1538) -> (x != y?=w1536:bool)
    n1359 = case shown="True" w1544 {
      frame False {
        w1550 = TRUE ("Visible")
        n1360 = property on="Port 1a" class="Bool (strict)"("Visible"=w1550) -> ()  [unwired: 2 in, 2 out]
        n1361 = property on="Port 3" class="Bool (strict)"("Visible"=w1550) -> ()  [unwired: 2 in, 2 out]
      }
      frame True {
        w1551 = TRUE ("Visible")
        n1362 = property on="Port 1a" class="Bool (strict)"("Visible"=w1551) -> ()  [unwired: 2 in, 2 out]
        n1363 = property on="Port 3" class="Bool (strict)"("Visible"=w1551) -> ()  [unwired: 2 in, 2 out]
      }
    }
    n1364 = Wait (ms)(milliseconds to wait=u32 40) -> ()  [unwired: 1 out]
    n1365 = case shown="True" w1536 {
      tunnel: [w1548 errorcluster {"status"=TRUE, "code"=0, "source"="Init"} ("error out")] -> w1537
      tunnel: w1540 -> [w1548 _]
      frame False {
      }
      frame True {
      }
    }
    n1366 = case shown="No Error" w1537 {
      selector: w1537 -> [w1558 w1585]
      tunnel: [w1561 w1589] -> w1547
      tunnel: [w1560 w1583] -> w1546
      tunnel: w1538 -> [w1559 w1587]
      frame No Error {
        n1367 = property class="Instr"(reference=w1559, error in=w1558) -> (reference out=w1556:refnum<visa-resource-name>, error out=w1557:errorcluster, "Serial Settings:Number of Bytes at Serial Port"=w1553:u32)
        n1368 = Greater?(x=w1553, y=u32 5) -> (0:w1552:bool)
        n1369 = Not(x=w1552) -> (.not. x?=→"Port 1a":bool)
        n1370 = while {
          tunnel: [w1578] -> w1560
          tunnel: [w1577] -> w1561
          tunnel: w1557 -> [w1576]
          tunnel: w1556 -> [w1575]
          stop <- TRUE stop-if-true
          n1371 = property class="Instr" props=["Serial Settings:Number of Bytes at Serial Port"](reference=w1575, error in=w1576) -> (reference out=w1580:refnum<visa-resource-name>, error out=w1579:errorcluster)  [unwired: 1 out]
          n1372 = VISA Read(VISA resource name=w1580, byte count=u32 50, error in (no error)=w1579) -> (VISA resource name out=w1577:refnum<visa-resource-name>, read buffer=w1562:string, error out=w1578:errorcluster)  [unwired: 1 out]
          "UNI READ" <- w1562
          n1373 = Spreadsheet String To Array(delimiter (Tab)=";", format string="", spreadsheet string=w1562, array type (2D Dbl)=dbl[] []) -> (array=w1572:dbl[])
          n1374 = Index Array(array=w1572) -> (element #1=→"LVDT MIN":dbl, element #2=→"LVDT MAX":dbl, element #3=→"LVDT Peak":dbl, element #4=→"pizo raw":dbl, element #5=→"Friction":dbl, element #6=→"cof 2":dbl)  [unwired: 6 in]
        }
      }
      frame Error {
        w1595 = u16 0 items=["None", "XON/XOFF", "RTS/CTS", "XON/XOFF & RTS/CTS", "DTR/DSR", "XON/XOFF & DTR/DSR"] ("flow control (0:none)  2")
        w1593 = u16 10 items=["1.0"=10, "1.5"=15, "2.0"=20] ("stop bits 2")
        w1591 = u16 0 items=["None", "Odd", "Even", "Mark", "Space"] ("parity 2")
        w1592 = u32 10000  # timeout (10sec)
        n1375 = VISA Close(VISA resource name=w1587, error in (no error)=w1585) -> (error out=w1588:errorcluster)
        n1376 = local write "Port 1a"(FALSE ("Port 1a")) -> ()
        n1377 = local read "Com Port 1"() -> (w1582:refnum<visa-resource-name>)
        n1378 = call <vilib>:"Clear Errors.vi"("error in (no error)"=w1588) -> ("error out"=w1586:errorcluster)  [unwired: 5 in, 1 out]
        n1379 = call-poly "VISA Configure Serial Port"("VISA resource name"=w1582, "timeout (10sec)"=w1592, "baud rate (9600)"=u32 250000 ("baud rate  2"), "data bits (8)"=u16 8 ("data bits  2"), "parity (0:none)"=w1591, "error in (no error)"=w1586, "stop bits (10: 1 bit)"=w1593, "flow control (0:none)"=w1595) -> ("VISA resource name out"=w1596:refnum<visa-resource-name>, "error out"=w1597:errorcluster)  [unwired: 6 in]
        n1380 = flat-sequence {
          tunnel: w1596 -> [w1599]
          tunnel: w1597 -> [w1598]
          tunnel: [w1599] -> w1589
          tunnel: [w1598] -> w1583
          frame #0 {
            n1381 = Wait (ms)(milliseconds to wait=u32 50) -> ()  [unwired: 1 out]
          }
        }
        "Residual Uno" <- ""
        "Port 1 Error" <- w1583
      }
    }
    n1382 = local read "Quit"() -> (w1535:bool)
    "Error Uno" <- w1540
  }
  n1383 = while {
    stop <- w1609 stop-if-true
    # "V0OLTAGE TO STROKE (peice vise calibration)"
    n1384 = Wait (ms)(milliseconds to wait=u32 10) -> ()  [unwired: 1 out]
    n1385 = local read "LVDT Peak"() -> (w1601:dbl)
    n1386 = formula code="// Dynamic Parameterized Linear Interpolation Node\n// Inputs: vpp_val, voltages (Array), distances (Array)\n// Outputs: stroke\n\nint i = 0;\nint segments = 11; // 12 points make 11 interpolation segments\n\n// 1. Lower Boundary Clamp\nif (vpp_val <= voltages[0]) {\n    stroke = distances[0];\n}\n// 2. Upper Boundary Clamp\nelse if (vpp_val >= voltages[segments]) {\n    stroke = distances[segments];\n}\n// 3. Dynamic Segment Search Loop\nelse {\n    stroke = distances[0]; // Fallback baseline\n    for (i = 0; i < segments; i++) {\n        if (vpp_val >= voltages[i] && vpp_val <= voltages[i+1]) {\n            // Standard linear interpolation formula using array lookups\n            stroke = distances[i] + (vpp_val - voltages[i]) * (distances[i+1] - distances[i]) / (voltages[i+1] - voltages[i]);\n            break; // Segment found, safely exit the loop\n        }\n    }\n}"("vpp_val"=w1601, "voltages"="calibration values", "distances"="STROKE") -> ("stroke"=→"LVDT STROKE":dbl)
    n1387 = local read "Calibration Tare Value"() -> (w1605:dbl)
    n1388 = local read "Calibration Tare"() -> (w1603:bool)
    n1389 = Subtract(x=w1601, y=w1605) -> (x-y=→"LVDT STROKE  Calibration":dbl)
    n1390 = case shown="True" w1603 {
      selector: w1603 -> [_ w1611]
      tunnel: w1601 -> [_ w1612]
      frame False {
      }
      frame True {
        n1391 = Not(x=w1611) -> (.not. x?=w1610:bool)
        n1392 = local write "Calibration Tare"(w1610) -> ()
        "Calibration Tare Value" <- w1612
      }
    }
    n1393 = local read "Quit"() -> (w1609:bool)
  }
  n1394 = while {
    stop <- w1632 stop-if-true
    n1395 = call <vilib>:"High Resolution Polling Wait.vi"("seconds to wait"=0.02) -> ()  [unwired: 10 in, 1 out]
    n1396 = local read "Due read"() -> (w1630:string)
    n1397 = Spreadsheet String To Array(delimiter (Tab)=";", format string="", spreadsheet string=w1630, array type (2D Dbl)=string[] []) -> (array=w1627:string[])
    n1398 = Fract/Exp String To Number(string=w1627) -> (number=w1626:dbl[])  [unwired: 3 in, 1 out]
    n1399 = Index Array(array=w1626) -> (element #1=→"Sample Temperature":dbl, element #2=→"Target Sample Temperature":dbl, element #3=→"Current Duty Cycle":dbl, element #4=→"Ambient Temperature":dbl, element #5=→"Dac Status":dbl, element #6=→"Vpp":dbl, element #7=→"Active Error Code":dbl, element #8=→"Kp":dbl, element #9=→"Ki":dbl, element #10=→"Kd":dbl, element #11=→"SampleRaw":dbl, element #12=→"AmbRaw":dbl)  [unwired: 12 in]
    n1400 = local read "Quit"() -> (w1632:bool)
  }
  n1401 = while {
    shift-right: [w1646] -> w37
    shift-left: _ -> [w1637]
    shift-right: [w1645] -> w36
    shift-left: errorcluster {"status"=FALSE, "code"=0, "source"="Init"} ("error out") -> [w1639]
    tunnel: [w1634] -> w41
    tunnel: [w1644] -> _
    i -> [w1644]
    stop <- w1634 stop-if-true
    n1402 = local read "Com Port 2"() -> (w1638:refnum<visa-resource-name>)
    n1403 = local read "Port 2a"() -> (w1640:bool)
    n1404 = Unbundle(w1639) -> ("status"=→"Port 4":bool)  [unwired: 2 out]
    n1405 = call <vilib>:"High Resolution Polling Wait.vi"("seconds to wait"=0.02) -> ()  [unwired: 10 in, 1 out]
    n1406 = local read "Port 4"() -> (w1641:bool)
    n1407 = Not Equal?(x=w1638, y=w1637) -> (x != y?=w1636:bool)
    n1408 = Or(x=w1641, y=w1640) -> (x .or. y?=w1643:bool)
    n1409 = case shown="False" w1643 {
      frame False {
        w1649 = TRUE ("Visible")
        n1410 = property on="Port 2a" class="Bool (strict)"("Visible"=w1649) -> ()  [unwired: 2 in, 2 out]
        n1411 = property on="Port 4" class="Bool (strict)"("Visible"=w1649) -> ()  [unwired: 2 in, 2 out]
      }
      frame True {
        w1650 = TRUE ("Visible")
        n1412 = property on="Port 2a" class="Bool (strict)"("Visible"=w1650) -> ()  [unwired: 2 in, 2 out]
        n1413 = property on="Port 4" class="Bool (strict)"("Visible"=w1650) -> ()  [unwired: 2 in, 2 out]
      }
    }
    n1414 = case shown="True" w1636 {
      tunnel: [w1647 errorcluster {"status"=TRUE, "code"=0, "source"="Init"} ("error out")] -> w1635
      tunnel: w1639 -> [w1647 _]
      frame False {
      }
      frame True {
      }
    }
    n1415 = case shown="Error" w1635 {
      selector: w1635 -> [w1662 w1694]
      tunnel: [w1655 w1699] -> w1646
      tunnel: [w1663 w1692] -> w1645
      tunnel: w1637 -> [w1665 w1697]
      frame No Error {
        n1416 = property class="Instr" props=["Serial Settings:Number of Bytes at Serial Port"](reference=w1665, error in=w1662) -> (reference out=w1656:refnum<visa-resource-name>, error out=w1661:errorcluster)  [unwired: 1 out]
        n1417 = while {
          tunnel: [w1673] -> w1657
          tunnel: [w1672] -> w1658
          tunnel: w1661 -> [w1671]
          tunnel: w1656 -> [w1670]
          tunnel: [w1669] -> _
          i -> [w1669]
          stop <- TRUE stop-if-true
          n1418 = property class="Instr" props=["Serial Settings:Number of Bytes at Serial Port"](reference=w1670, error in=w1671) -> (reference out=w1675:refnum<visa-resource-name>, error out=w1674:errorcluster)  [unwired: 1 out]
          n1419 = VISA Read(VISA resource name=w1675, byte count=u32 1000, error in (no error)=w1674) -> (VISA resource name out=w1672:refnum<visa-resource-name>, read buffer=→"Due read":string, error out=w1673:errorcluster)  [unwired: 1 out]
        }
        n1420 = local read "Command"() -> (w1653:string)
        n1421 = call <vilib>:"Trim Whitespace.vi"("string"=w1653) -> ("trimmed string"=w1652:string)  [unwired: 1 in]
        n1422 = Not Equal?(x=w1652, y="") -> (x != y?=w1659:bool)
        n1423 = case shown="True" w1659 {
          tunnel: w1658 -> [w1677 w1682]
          tunnel: [w1677 w1686] -> w1664
          tunnel: w1657 -> [w1676 w1681]
          tunnel: [w1676 w1684] -> w1663
          tunnel: w1652 -> [_ w1680]
          tunnel: [_ w1683] -> _
          frame False {
            # "DATA  WRITE LOOP"
          }
          frame True {
            n1424 = Concatenate Strings(w1680, "\r\n") -> (w1679:string)
            n1425 = VISA Write(VISA resource name=w1682, write buffer=w1679, error in (no error)=w1681) -> (VISA resource name out=w1686:refnum<visa-resource-name>, return count=w1683:u32, error out=w1685:errorcluster)
            n1426 = flat-sequence {
              tunnel: w1685 -> [w1688]
              tunnel: [w1688] -> w1684
              frame #0 {
                n1427 = local write "Command"("" ("Command")) -> ()
                n1428 = Wait (ms)(milliseconds to wait=u32 5) -> ()  [unwired: 1 out]
              }
            }
          }
        }
        n1429 = VISA Flush I/O Buffer(VISA resource name=w1664) -> (VISA resource name out=w1655:refnum<visa-resource-name>, error out=→"error out 9":errorcluster)  [unwired: 2 in]
        "Port 2a" <- TRUE ("Port 2a")
      }
      frame Error {
        w1705 = u16 0 items=["None", "XON/XOFF", "RTS/CTS", "XON/XOFF & RTS/CTS", "DTR/DSR", "XON/XOFF & DTR/DSR"] ("flow control (0:none)  2")
        w1703 = u16 10 items=["1.0"=10, "1.5"=15, "2.0"=20] ("stop bits 2")
        w1701 = u16 0 items=["None", "Odd", "Even", "Mark", "Space"] ("parity 2")
        w1702 = u32 10000  # timeout (10sec)
        n1430 = VISA Clear(VISA resource name=w1697, error in (no error)=w1694) -> (VISA resource name out=w1696:refnum<visa-resource-name>, error out=w1695:errorcluster)
        n1431 = VISA Close(VISA resource name=w1696, error in (no error)=w1695) -> (error out=w1698:errorcluster)
        n1432 = call <vilib>:"Clear Errors.vi"("error in (no error)"=w1698) -> ()  [unwired: 5 in, 2 out]
        n1433 = local write "Port 2a"(FALSE ("Port 2a")) -> ()
        n1434 = local read "Com Port 2"() -> (w1691:refnum<visa-resource-name>)
        "visa due" <- w1691
        n1435 = call-poly "VISA Configure Serial Port"("VISA resource name"=w1691, "timeout (10sec)"=w1702, "baud rate (9600)"=u32 250000 ("baud rate  2"), "data bits (8)"=u16 8 ("data bits  2"), "parity (0:none)"=w1701, "stop bits (10: 1 bit)"=w1703, "flow control (0:none)"=w1705) -> ("VISA resource name out"=w1706:refnum<visa-resource-name>, "error out"=w1707:errorcluster)  [unwired: 7 in]
        n1436 = flat-sequence {
          tunnel: w1706 -> [w1709]
          tunnel: w1707 -> [w1708]
          tunnel: [w1709] -> w1699
          tunnel: [w1708] -> w1692
          frame #0 {
            n1437 = Wait (ms)(milliseconds to wait=u32 50) -> ()  [unwired: 1 out]
          }
        }
        "Residual Due" <- ""
        "Port 2 Error" <- w1692
      }
    }
    n1438 = local read "Quit"() -> (w1634:bool)
    "Error Due" <- w1639
  }
  n1439 = local write "FRICVALZ"(0.0 ("FRICVALZ")) -> ()
  n1440 = property on="RUN" class="Bool (strict)"("Visible"=TRUE) -> ()  [unwired: 2 in, 2 out]
  n1441 = while {
    tunnel: [w1726] -> _
    tunnel: [w1711] -> w54
    i -> [w1726]
    stop <- w1711 stop-if-true
    n1442 = local read "conststatus"() -> (w1715:dbl)
    n1443 = local read "Main Tab"() -> (w1713:T2)
    n1444 = local read "EDIT"() -> (w1732:bool)
    n1445 = local read "Rate"() -> (w1731:dbl)
    n1446 = case shown="True" w1732 {
      tunnel: [FALSE TRUE] -> w1718
      frame False {
      }
      frame True {
      }
    }
    n1447 = property on="Time slide" class="Slide (strict)"("Scale.Range:Maximum"=2500.0) -> ()  [unwired: 2 in, 2 out]
    n1448 = Equal?(x=w1713, y=T26."About" ("Main Tab")) -> (x = y?=w1724:bool)
    n1449 = Equal?(x=w1715, y=0.0) -> (x = y?=w1716:bool)
    n1450 = Divide(x=1.0, y=w1731) -> (x/y=w1727:dbl)
    "Time 2" <- w1727
    n1451 = case shown="True" w1716 {
      frame False {
      }
      frame True {
        # "C:\\WinDucom\\calibrate WO 2391.dcf"
        n1452 = local write "Lan flag"(22) -> ()
        n1453 = local write "conststatus"(10.0 ("rpm value : 2")) -> ()
        n1454 = String To Path(string="C:\\LAB-IQ\\calibrate WO 2465.dcf") -> (path=w1738:path)
        n1455 = Open/Create/Replace File "Open File"(file path (use dialog)=w1738) -> (refnum out=w1736:refnum<file>)  [unwired: 5 in, 2 out]
        n1456 = for {
          N: 23 -> [_]
          tunnel: w1736 -> [w1747]
          i -> [w1741]
          (unwired) TRUE ("line mode (F)")
          n1457 = Read from Text File "Read File"(file (use dialog)=w1747) -> (text=w1746:string)  [unwired: 3 in, 3 out]
          n1458 = Match Pattern(string=w1746, regular expression="]") -> (after substring=w1744:string)  [unwired: 1 in, 3 out]
          n1459 = String Subset(string=w1746, offset (0)=5, length (rest)=10 ("length (rest)")) -> (substring=w1739:string)
          n1460 = Fract/Exp String To Number(string=w1739) -> (number=w1740:dbl)  [unwired: 3 in, 1 out]
          n1461 = Match Pattern(string=w1744, regular expression="-") -> (before substring=w1742:string)  [unwired: 1 in, 3 out]
          n1462 = case shown="4" w1741 {
            tunnel: w1740 -> [w1750 w1751 w1752 w1753 _ _ _ w1758 w1759 _ w1760 w1761 w1762 w1763 w1764 w1765 _ w1766 w1767 _ _ _ _ _]
            tunnel: w1742 -> [_ _ _ _ w1754 w1755 w1756 _ _ _ _ _ _ _ _ _ _ _ _ w1768 w1769 w1770 w1771 _]
            frame 0 {
              n1463 = local write "FRIC. FORCE :"(w1750) -> ()
            }
            frame 1 {
              n1464 = local write "TEMPERATURE :"(w1751) -> ()
            }
